vi "WorksheetName_toStringArray.vi"(8 "error in (no error)":errorcluster, 10 "Worksheet Index":string, 11 "ExcelFile in":refnum<class "PortableExcelFileManipulationOXML.lvclass">) -> (0 "error out":errorcluster, 2 "Array":string[][](array[string]), 3 "ExcelFile out":refnum<class "PortableExcelFileManipulationOXML.lvclass">)   [LabVIEW 2019, in "PortableExcelFileManipulationOXML.lvclass"]
doc: "This Function Takes an index to a spreadsheet as an input, and returns an 2d Array of strings from the index choosen."
uses:
  PortableExcelFileManipulationOXML.lvclass
  PortableExcelFileManipulationOXML.lvclass/PortableExcelFileManipulationOXML.ctl
  H:/LV projects/ExpressionEvaluator/Excel/ExcelManipulation.dll
  ExcelManipulation.dll
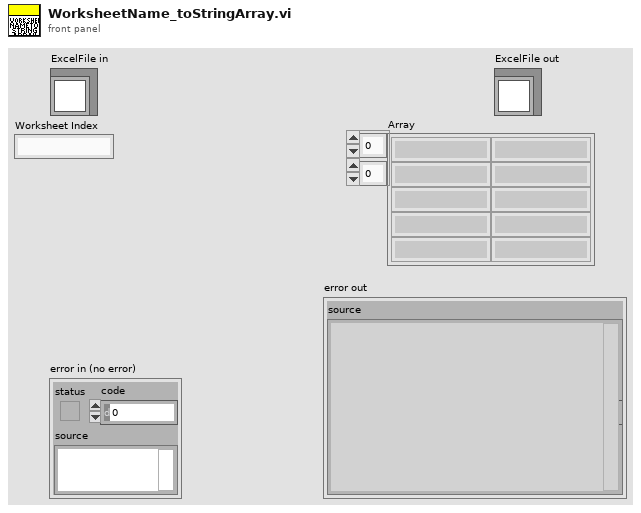
[diagram p1: front panel]
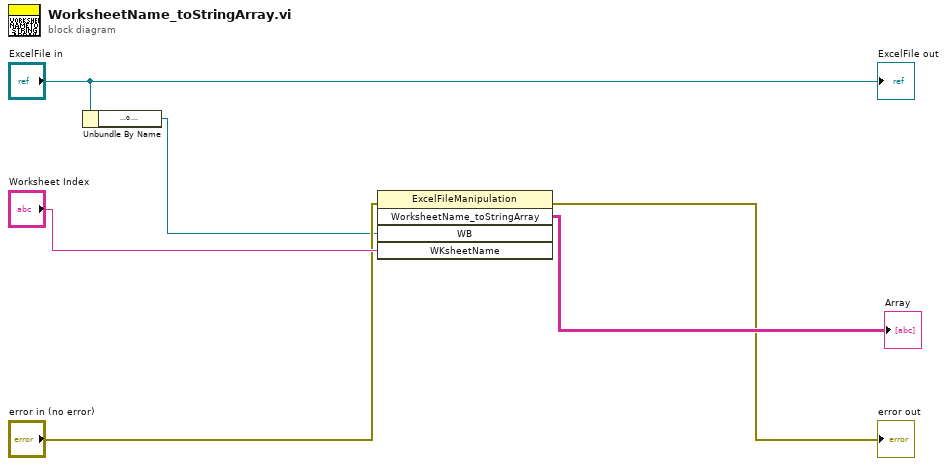
[diagram p0: block diagram]
diagram:
  n1 = Unbundle By Name("ExcelFile in") -> ("ExcelOpen"=w1:refnum<k24>)
  n2 = invoke class="ExcelFileManipulation" method="WorksheetName_toStringArray"(error in="error in (no error)", "WB"=w1, "WKsheetName"="Worksheet Index") -> (error out=→"error out":errorcluster, "WorksheetName_toStringArray"=→"Array":string[][])  [unwired: 2 in, 3 out]
  "ExcelFile out" <- "ExcelFile in"
